vi "Event Handler.vi"(8 "error in (no error)":errorcluster, 11 "Component.JSONEditor in":refnum<class "Component.JSONEditor.lvclass">) -> ()   [LabVIEW 2021, in "Component.JSONEditor.lvclass"]
uses:
  Component.JSONEditor.lvclass
  E:/Git/WebView-Components/Source/Component_class/Component.lvclass
  Component.JSONEditor.lvclass/Component.JSONEditor.ctl
  private/JSON Updated Event Data--cluster.ctl
  e3f92d98-e7ad-4bc2-98b6-bd4194dccb6e.vi
  <vilib>/sklein/WebView2/Webview2 Lib/WebView2 Control Object/Read Events.vi
  <vilib>/JDP Science/JSONtext/Next JSON Value.vi
  <vilib>/JDP Science/JSONtext/String Subset.vi
  <vilib>/JDP Science/JSONtext/Parsing/Advance past next JSON Value (inlined COPY).vi
  <vilib>/JDP Science/JSONtext/Parsing/Advance past whitespace.vi
  <vilib>/JDP Science/JSONtext/Parsing/Advance past String.vi
  <vilib>/JDP Science/JSONtext/Parsing/Advance past Number.vi
  <vilib>/JDP Science/JSONtext/Parsing/Advance past Line Ending.vi
  <vilib>/sklein/WebView2/Webview2 Lib/WebView2 Control Object/Register Events.vi
  <vilib>/JDP Science/JSONtext/Parsing/Parse Full Path or Item Name.vi
  <vilib>/JDP Science/JSONtext/Parsing/Advance past Array.vi
  <vilib>/JDP Science/JSONtext/Parsing/Advance past Object.vi
  <vilib>/JDP Science/JSONtext/support/Error Cluster From Code.vi
  <vilib>/JDP Science/JSONtext/Offset/Find Item Locations by Path.vi
  <vilib>/JDP Science/JSONtext/JSON text to Variant.vi
  <vilib>/sklein/WebView2/Webview2 Lib/WebView2 Control Object/WebView2 Control.lvclass
  <vilib>/JDP Science/JSONtext/LVClass Serializer/JSONtext LVClass Serializer.lvclass
  <vilib>/JDP Science/JSONtext/JSONtext.lvlib
  Component_class/Component.lvclass
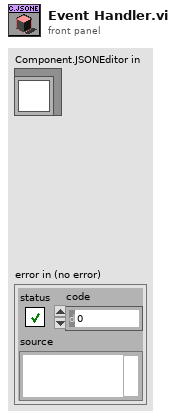
[diagram p1: front panel]
types:
  T1 = typedef "Component.JSONEditor.lvclass/JSONEditor Events.ctl" = cluster{"JSON Updated":refnum<user-event>, "Selected Node Path":refnum<user-event>}
  T2 = typedef "WebView2.lvlib/WebView2 Control.lvclass/Events.ctl" = cluster{"Navigation Complete Event":refnum<user-event>, "Source Changed Event":refnum<user-event>, "Document Title Changed Event":refnum<user-event>, "Status Bar Text Changed":refnum<user-event>, "Web Message Received":refnum<user-event>, "Window Close Requested":refnum<user-event>, "DOM Loaded":refnum<user-event>, "Navigation Started Event":refnum<user-event>}
  T3 = typedef "Component.JSONEditor.lvclass/JSON Updated Event Data--cluster.ctl" = cluster{"JSON":string}
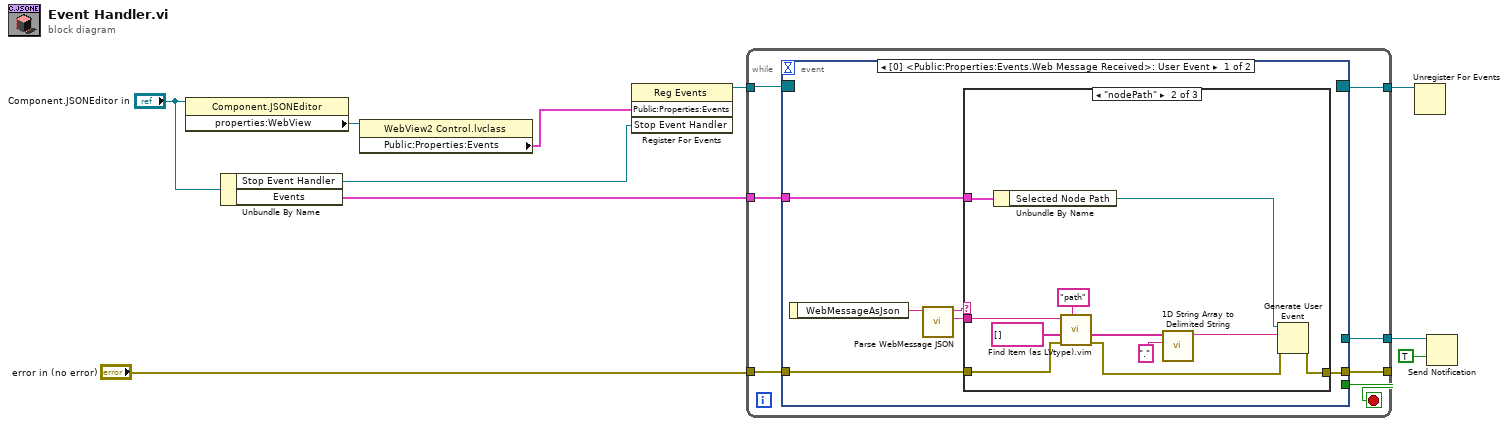
[diagram p0: block diagram]
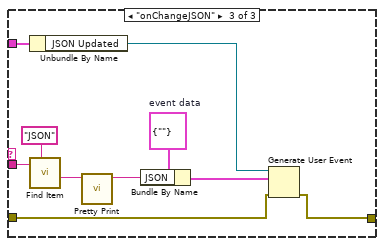
[diagram p3: hidden frame]
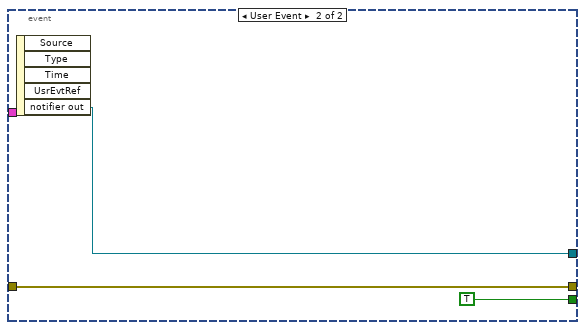
[diagram p4: hidden frame]
diagram:
  n1 = property class="Component.JSONEditor"(reference="Component.JSONEditor in") -> ("properties:WebView"=w2:refnum<class "WebView2 Control.lvclass">)  [unwired: 1 in, 2 out]
  n2 = Unbundle By Name("Component.JSONEditor in") -> ("Stop Event Handler"=w7:refnum<user-event>, "Events"=w5:T1)
  n3 = property class="WebView2 Control.lvclass"(reference=w2) -> ("Public:Properties:Events"=w1:T2)  [unwired: 1 in, 2 out]
  n4 = register-events(w1, w7) -> (reference out=w9:refnum<event-registration>)  [unwired: 2 in, 1 out]
  n5 = while {
    tunnel: w9 -> [w13]
    tunnel: [w17] -> _
    tunnel: "error in (no error)" -> [w16]
    tunnel: [w14] -> w10
    tunnel: w5 -> [w12]
    tunnel: [w11] -> w4
    stop <- w15 stop-if-true
    n6 = event shown="[0] <Public:Properties:Events.Web Message Received>: User Event" {
      selector: w13 -> [_ _]
      dyn-events: [_ _] -> w14
      timeout: _ -> [_ _]
      tunnel: [w19 w48] -> w17
      tunnel: w16 -> [w20 w48]
      tunnel: [_ TRUE] -> w15
      tunnel: w12 -> [w18 _]
      tunnel: [_ w46] -> w11
      event User Event {
        n7 = event-data() -> ("WebMessageAsJson"=w23:string)  [unwired: 1 in]
        n8 = call "Parse WebMessage JSON.vi"("JSON in"=w23) -> ("Data out"=w21:string, "Type out"=w22:string)  [unwired: 9 in]
        n9 = case shown="\"nodePath\"" w22 {
          tunnel: w21 -> [_ w35 w41]
          tunnel: w20 -> [w24 w34 w42]
          tunnel: [w24 w28 w43] -> w19
          tunnel: w18 -> [_ w31 w45]
          frame Default {
          }
          frame "nodePath" {
            n10 = Unbundle By Name(w31) -> ("Selected Node Path"=w30:refnum<user-event>)
            n11 = call "Find Item (as LVtype).vim"("$Path or Item Name"="path", "error in (no error)"=w34, "Data Type and Default Value"=string[] [], "JSON"=w35) -> ("error out"=w29:errorcluster, "Data"=w26:string[])  [unwired: 4 in, 2 out]
            n12 = call <vilib>:"1D String Array to Delimited String.vi"("delimiter"=".", "string array"=w26) -> ("delimited string"=w25:string)  [unwired: 9 in]
            n13 = Generate User Event(user event=w30, event data cluster=w25, error in=w29) -> (error out=w28:errorcluster)  [unwired: 1 in, 1 out]
          }
          frame "onChangeJSON" {
            w40 = T3 {"JSON"=""}  # event data
            n14 = Unbundle By Name(w45) -> ("JSON Updated"=w44:refnum<user-event>)
            n15 = call <vilib>:"Find Item.vi"("$Path or Item Name"="JSON", "JSON"=w41) -> ("<JSON>"=w38:string)  [unwired: 6 in, 3 out]
            n16 = call <vilib>:"Pretty Print.vi"("JSON"=w38) -> ("<JSON>"=w36:string)  [unwired: 8 in, 2 out]
            n17 = Bundle By Name(cluster=w40, "JSON"=w36) -> (w39:T3)
            n18 = Generate User Event(user event=w44, event data cluster=w39, error in=w42) -> (error out=w43:errorcluster)  [unwired: 1 in, 1 out]
          }
        }
      }
      event User Event {
        n19 = event-data() -> ("notifier out"=w46:refnum<notifier>)  [unwired: 1 in, 4 out]
      }
    }
  }
  n20 = Unregister For Events(event registration refnum=w10) -> ()  [unwired: 1 in, 1 out]
  n21 = Send Notification(notification=TRUE, notifier=w4) -> ()  [unwired: 1 in, 2 out]
